vi "Create DAQmx Channels.vi"(8 "error in (no error)":errorcluster, 10 "Channels":refnum<class "Channel Config.lvclass">[](array[class])) -> (0 "error out":errorcluster, 2 "DAQmxChannels":refnum<class "DAQmxChannel.lvclass">[](array[class]))   [LabVIEW 2023, in "VolatusDAQConfig.lvlib"]
uses:
  VolatusDAQConfig.lvlib
  DAQmxChannel/DAQmxChannel.lvclass
  VolatusConfig/VolatusConfigElement/VolatusConfigElement.lvclass/VolatusConfigElement.ctl
  DAQmxVoltageChannel/VoltageInChannel.lvclass
  VoltageOutChannel/VoltageOutChannel.lvclass
  CurrentInChannel/CurrentInChannel.lvclass
  CurrentOutChannel/CurrentOutChannel.lvclass
  DAQmxThermocoupleChannel/TCChannel.lvclass
  RTDChannel/RTDChannel.lvclass
  IEPEChannel/IEPEChannel.lvclass
  DigitalOutChannel/DigitalOutChannel.lvclass
  DigitalInChannel/DigitalInChannel.lvclass
  BridgeChannel/BridgeChannel.lvclass
  lv-cdm/CDM-Config/Config Lookup/Match Meta.vi
  lv-cdm/CDM-Config/Config Element/Owner.vi
  lv-cdm/CDM-Config/Config Manager/Lookup Descendant.vi
  lv-cdm/CDM-Config/Config Filter/Config Lookup.lvclass
  lv-cdm/CDM-Config/Config Element/Config Element.lvclass
  VolatusConfig/VolatusConfigElement/VolatusConfigElement.lvclass
  StrainChannel/StrainChannel.lvclass
  C:/dev/volatus/mts-volatus-super/libs/lv-volatus/VolatusConfig/Channel/Channel Config.lvclass
  C:/dev/volatus/mts-volatus-super/libs/lv-volatus/VolatusConfig/VolatusConfigElement/VolatusConfigElement.lvclass
  C:/dev/volatus/mts-volatus-super/libs/lv-volatus/VolatusDAQConfig/DAQmxChannel/DAQmxChannel.lvclass
  VolatusConfig/Channel/Channel Config.lvclass
  C:/dev/volatus/mts-volatus-super/libs/lv-volatus/VolatusDAQConfig/DAQmxVoltageChannel/VoltageInChannel.lvclass
  C:/dev/volatus/mts-volatus-super/libs/lv-volatus/VolatusDAQConfig/VoltageOutChannel/VoltageOutChannel.lvclass
  C:/dev/volatus/mts-volatus-super/libs/lv-volatus/VolatusDAQConfig/CurrentInChannel/CurrentInChannel.lvclass
  C:/dev/volatus/mts-volatus-super/libs/lv-volatus/VolatusDAQConfig/CurrentOutChannel/CurrentOutChannel.lvclass
  C:/dev/volatus/mts-volatus-super/libs/lv-volatus/VolatusDAQConfig/DAQmxThermocoupleChannel/TCChannel.lvclass
  C:/dev/volatus/mts-volatus-super/libs/lv-volatus/VolatusDAQConfig/RTDChannel/RTDChannel.lvclass
  C:/dev/volatus/mts-volatus-super/libs/lv-volatus/VolatusDAQConfig/IEPEChannel/IEPEChannel.lvclass
  C:/dev/volatus/mts-volatus-super/libs/lv-volatus/VolatusDAQConfig/DigitalOutChannel/DigitalOutChannel.lvclass
  C:/dev/volatus/mts-volatus-super/libs/lv-volatus/VolatusDAQConfig/DigitalInChannel/DigitalInChannel.lvclass
  C:/dev/volatus/mts-volatus-super/libs/lv-volatus/VolatusDAQConfig/BridgeChannel/BridgeChannel.lvclass
  C:/dev/volatus/mts-volatus-super/libs/lv-volatus/VolatusDAQConfig/StrainChannel/StrainChannel.lvclass
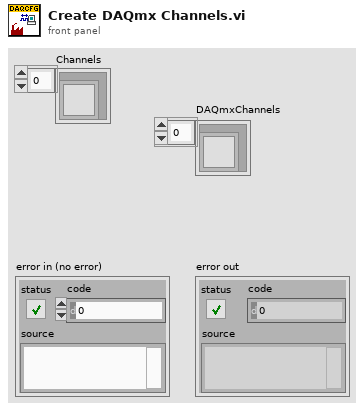
[diagram p1: front panel]
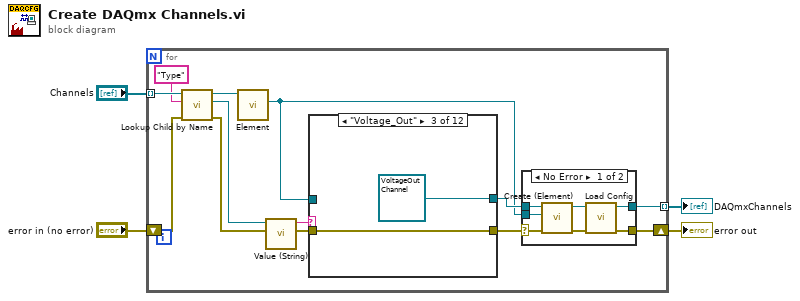
[diagram p0: block diagram]
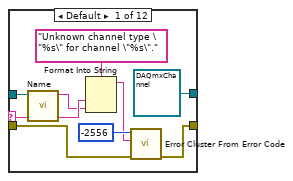
[diagram p3: hidden frame]
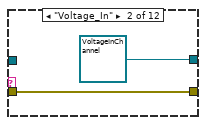
[diagram p4: hidden frame]
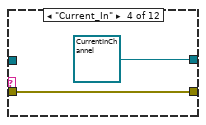
[diagram p5: hidden frame]
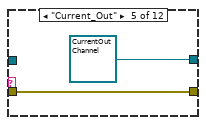
[diagram p6: hidden frame]
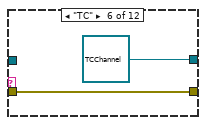
[diagram p7: hidden frame]
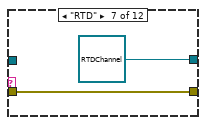
[diagram p8: hidden frame]
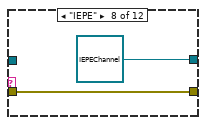
[diagram p9: hidden frame]
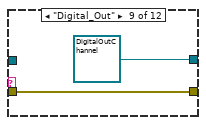
[diagram p10: hidden frame]
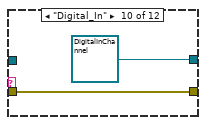
[diagram p11: hidden frame]
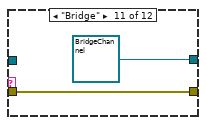
[diagram p12: hidden frame]
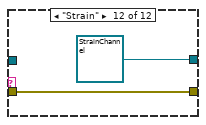
[diagram p13: hidden frame]
diagram:
  n1 = for {
    tunnel: "Channels" -> [w16] mode=indexing
    shift-right: [w11] -> w1
    shift-left: "error in (no error)" -> [w17]
    tunnel: [w10] -> w4 mode=indexing
    n2 = call "Lookup Child by Name.vi"("error in (no error)"=w17, "Child Name"="Type" ("Name"), "VolatusConfigElement in"=w16) -> ("error out"=w14:errorcluster, "Child"=w7:refnum<class "Config Element.lvclass">, "VolatusConfigElement out"=w6:refnum<class "Channel Config.lvclass">)  [unwired: 5 in, 1 out]
    n3 = call "Element.vi"("VolatusConfigElement in"=w6) -> ("Element"=w5:refnum<class "Config Element.lvclass">)  [unwired: 9 in, 1 out]
    n4 = call "Value (String).vi"("error in (no error)"=w14, "Config Element in"=w7) -> ("error out"=w12:errorcluster, "String Value"=w13:string)  [unwired: 8 in]
    n5 = case shown="\"Voltage_Out\"" w13 {
      selector: w13 -> [w32 _ _ _ _ _ _ _ _ _ _ _]
      tunnel: w12 -> [w34 w36 w38 w40 w42 w44 w46 w48 w50 w52 w54 w55]
      tunnel: [w28 w36 w38 w40 w42 w44 w46 w48 w50 w52 w54 w55] -> w9
      tunnel: w5 -> [w27 _ _ _ _ _ _ _ _ _ _ _]
      tunnel: [refnum<class "DAQmxChannel.lvclass"> refnum ("VolatusDAQConfig:DAQmxThermocoupleChannel") refnum<class "VoltageInChannel.lvclass"> refnum ("VolatusDAQConfig:DAQmxVoltageChannel.lvclass") refnum<class "VoltageOutChannel.lvclass"> refnum ("VolatusDAQConfig:VoltageOutChannel.lvclass") refnum<class "CurrentInChannel.lvclass"> refnum ("VolatusDAQConfig:CurrentInChannel.lvclass") refnum<class "CurrentOutChannel.lvclass"> refnum ("VolatusDAQConfig:CurrentOutChannel.lvclass") refnum<class "TCChannel.lvclass"> refnum ("VolatusDAQConfig:DAQmxThermocoupleChannel") refnum<class "RTDChannel.lvclass"> refnum ("VolatusDAQConfig:RTDChannel.lvclass") refnum<class "IEPEChannel.lvclass"> refnum ("VolatusDAQConfig:IEPEChannel.lvclass") refnum<class "DigitalOutChannel.lvclass"> refnum ("VolatusDAQConfig:DigitalOutChannel.lvclass") refnum<class "DigitalInChannel.lvclass"> refnum ("VolatusDAQConfig:DigitalInChannel.lvclass") refnum<class "BridgeChannel.lvclass"> refnum ("VolatusDAQConfig:BridgeChannel.lvclass") refnum<class "StrainChannel.lvclass"> refnum ("VolatusDAQConfig:StrainChannel.lvclass")] -> w8
      frame Default {
        n6 = call "Name.vi"("Config Element in"=w27) -> ("Name"=w29:string)  [unwired: 9 in, 1 out]
        n7 = Format Into String(format string="Unknown channel type \"%s\" for channel \"%s\".", w32, w29) -> (resulting string=w31:string)  [unwired: 2 in, 1 out]
        n8 = call <vilib>:"Error Cluster From Error Code.vi"("error in (no error)"=w34, "error message (\"\")"=w31, "error code (0)"=-2556) -> ("error out"=w28:errorcluster)  [unwired: 6 in]
      }
      frame "Voltage_In" {
      }
      frame "Voltage_Out" {
      }
      frame "Current_In" {
      }
      frame "Current_Out" {
      }
      frame "TC" {
      }
      frame "RTD" {
      }
      frame "IEPE" {
      }
      frame "Digital_Out" {
      }
      frame "Digital_In" {
      }
      frame "Bridge" {
      }
      frame "Strain" {
      }
    }
    n9 = case shown="No Error" w9 {
      selector: w9 -> [w21 w25]
      tunnel: [w24 w25] -> w11
      tunnel: [w23 _] -> w10
      tunnel: w8 -> [w20 _]
      tunnel: w5 -> [w19 _]
      frame No Error {
        n10 = call "Create (Element).vi"("error in (no error)"=w21, "Element"=w19, "VolatusConfigElement in"=w20) -> ("error out"=w22:errorcluster, "VolatusConfigElement out"=w18:refnum<class "DAQmxChannel.lvclass">)  [unwired: 7 in]
        n11 = call-dynamic "Load Config.vi"("error in (no error)"=w22, "DAQmxChannel in"=w18) -> ("error out"=w24:errorcluster, "DAQmxChannel out"=w23:refnum<class "DAQmxChannel.lvclass">)  [unwired: 8 in]
      }
      frame Error {
      }
    }
  }
  "error out" <- w1
  "DAQmxChannels" <- w4
